vi "HD_Device in Use(Single).vi"(8 "error in (no error)":errorcluster, 9 "Alias":string, 10 "Selected Device":variant, 11 "temporary variable In":T1 {"Hardware Handle"."AWG"."Handle" format="0x%08x"; "Hardware Handle"."AWG"."Conn" format="0x%08x"; "Hardware Handle"."LIA"."Handle" format="0x%08x"; "Hardware Handle"."LIA"."Conn" format="0x%08x"; "Hardware Handle"."LIA DAQ Mod"."ModHandle" format="0x%08x"; "Hardware Handle"."LIA DAQ Mod"."Conn" format="0x%08x"}) -> (0 "error out":errorcluster, 3 "temporary variable Out":T1 {"Hardware Handle"."AWG"."Handle" format="0x%08x"; "Hardware Handle"."AWG"."Conn" format="0x%08x"; "Hardware Handle"."LIA"."Handle" format="0x%08x"; "Hardware Handle"."LIA"."Conn" format="0x%08x"; "Hardware Handle"."LIA DAQ Mod"."ModHandle" format="0x%08x"; "Hardware Handle"."LIA DAQ Mod"."Conn" format="0x%08x"})   [LabVIEW 2016, in "General.lvlib"]
uses:
  General.lvlib
  Main_Sweep_TemporaryVariable.ctl
  Main_Sweep_TemporaryVariable_Hardware.ctl
  Hardware_DeviceAddresses.ctl
  MW_ctl_DeviceHandles..ctl
  <instrlib>/Zurich Instruments LabOne/Public/ziTypeHandle.ctl
  <instrlib>/Zurich Instruments LabOne/Public/Modules/ziTypeModHandle.ctl
  Main_Sweep_TemporaryVariable_Data.ctl
  MW_ctl_Souce Freq..ctl
  <instrlib>/Zurich Instruments LabOne/Zurich Instruments LabOne.lvlib
  Microwave Source.lvlib
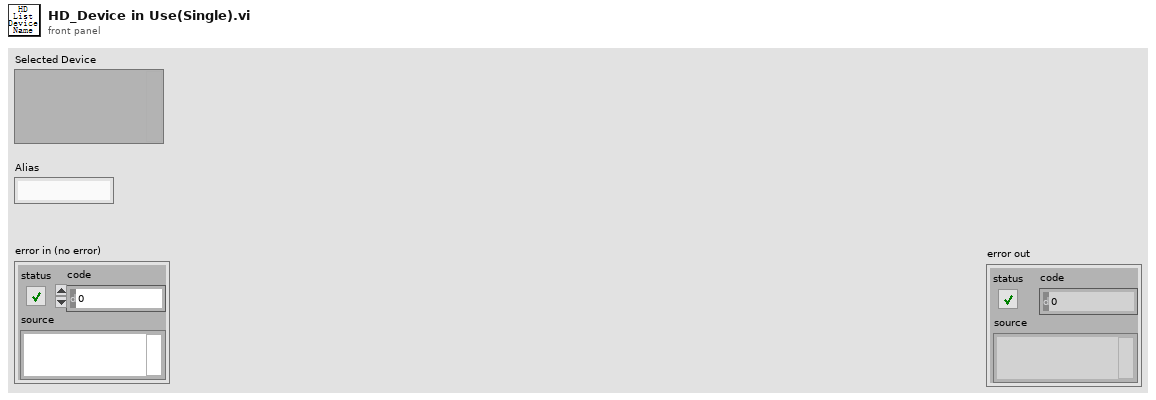
[diagram p1: front panel]
types:
  T1 = typedef "Main_Sweep_TemporaryVariable.ctl" = cluster{"Hardware Handle":T2, "Data":T7}
  T2 = typedef "Main_Sweep_TemporaryVariable_Hardware.ctl" = cluster{"Dev Add":T3, "AWG":T5, "LIA":T5, "LIA DAQ Mod":T6, "Devices in Use":string[][]}
  T3 = typedef "Hardware_DeviceAddresses.ctl" = cluster{"ZI Device Name":string[][], "MW Source":T4, "Trigger Delayer VISA":refnum<visa-resource-name>}
  T4 = typedef "Microwave Source.lvlib/MW_ctl_DeviceHandles..ctl" = cluster{"LO VISA":refnum<visa-resource-name>, "Probe VISA":refnum<visa-resource-name>, "Qubits":refnum<visa-resource-name>[]}
  T5 = typedef "Zurich Instruments LabOne.lvlib/ziTypeHandle.ctl" = cluster{"handleValid":bool, "Conn":u64, "Path Prefix":string, "Handle":u64, "Connected":bool, "Clockbase(s)":dbl}
  T6 = typedef "Zurich Instruments LabOne.lvlib/ziTypeModHandle.ctl" = cluster{"handleValid":bool, "Conn":u64, "ModHandle":u64, "moduleID":string, "Path Prefix":string}
  T7 = typedef "Main_Sweep_TemporaryVariable_Data.ctl" = cluster{"Demod R#1":dbl[][], "MW Source Freq":T8, "AWG PulseLength":cluster{"start":dbl, "step":dbl, "end":dbl, "iteration":dbl}, "Sweep Para.":cluster{"Sweep Para.":dbl[], "Sweep Readings":dbl[]}}
  T8 = typedef "Microwave Source.lvlib/MW_ctl_Souce Freq..ctl" = cluster{"start":dbl, "step":dbl, "end":dbl, "iteration":dbl, "diff":dbl}
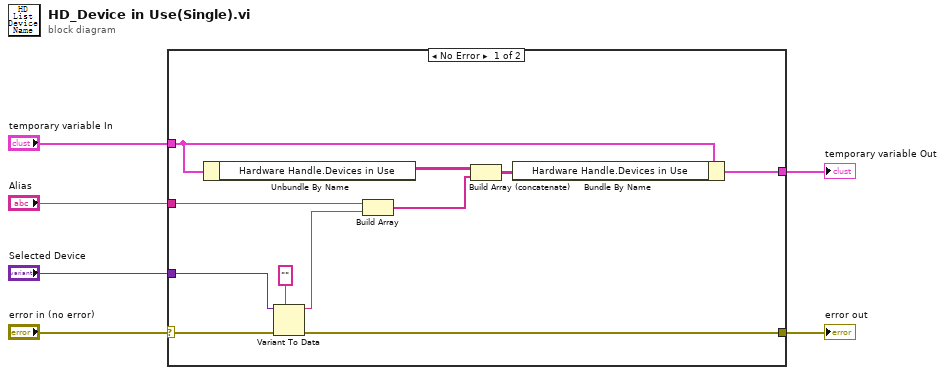
[diagram p0: block diagram]
diagram:
  n1 = case shown="No Error" "error in (no error)" {
    selector: "error in (no error)" -> [w7 w18]
    tunnel: "Alias" -> [w17 _]
    tunnel: "Selected Device" -> [w16 _]
    tunnel: [w13 w18] -> w4
    tunnel: [w12 w19] -> w3
    tunnel: "temporary variable In" -> [w11 w19]
    frame No Error {
      n2 = Unbundle By Name(w11) -> ("Hardware Handle.Devices in Use"=w10:string[][])
      n3 = Variant To Data(error in=w7, type="", Variant=w16) -> (data=w14:string, error out=w13:errorcluster)
      n4 = Build Array(w17, w14) -> (w8:string[])
      n5 = Build Array (concatenate)(w10, w8) -> (w9:string[][])
      n6 = Bundle By Name(cluster=w11, "Hardware Handle.Devices in Use"=w9) -> (w12:T1)
    }
    frame Error {
    }
  }
  "error out" <- w4
  "temporary variable Out" <- w3
